vi "Grid ChangeValue.vi"(8 "error in (no error)":errorcluster caption="エラー入力（エラーなし）", 9 "OldVal":string[][](array[string]), 10 "NewVal":string[][](array[string]), 11 "出力クラスタ":T2) -> (0 "error out":errorcluster caption="エラー出力", 2 "編集位置":T1, 3 "変化位置配列":T1[](array[typedef]))   [LabVIEW 2014]
uses:
  <vilib>/Utility/miscctls.llb/LVRowAndColumnTypeDef.ctl
  Grid Parameter.ctl
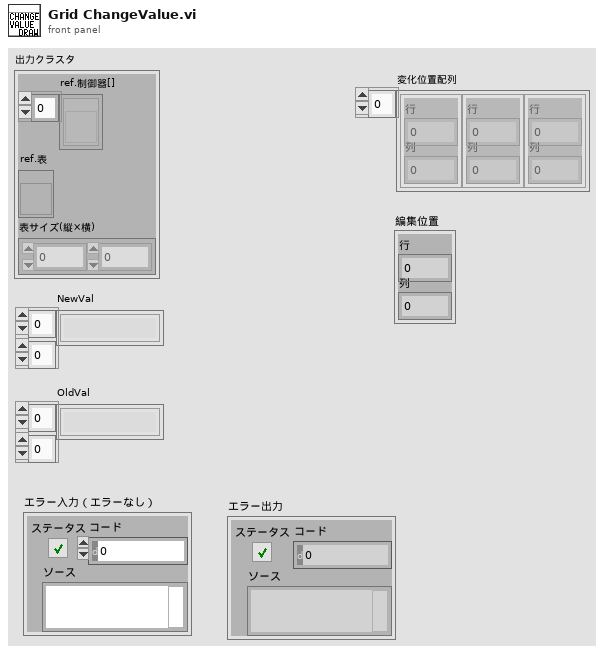
[diagram p1: front panel]
types:
  T1 = typedef "LVRowAndColumnTypeDef.ctl" = cluster{"Row":i32, "Column":i32}
  T2 = typedef "Grid Parameter.ctl" = cluster{"ref.制御器[]":refnum<vi>[], "ref.表":refnum<vi>, "表サイズ(縦×横)":i32[]}
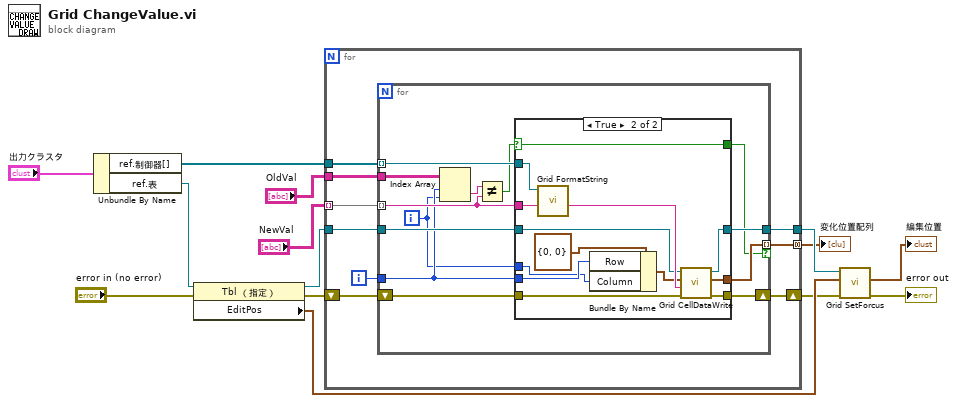
[diagram p0: block diagram]
diagram:
  n1 = Unbundle By Name("出力クラスタ") -> ("ref.制御器[]"=w2:refnum<vi>[], "ref.表"=w14:refnum<vi>)
  n2 = property class="Tbl （指定）"(reference=w14, error in="error in (no error)") -> (reference out=w10:refnum<vi>, error out=w1:errorcluster, "EditPos"=w12:T1)
  n3 = for {
    tunnel: "OldVal" -> [w23]
    tunnel: "NewVal" -> [w22] mode=indexing
    tunnel: w10 -> [w20]
    tunnel: [w19] -> w11
    shift-right: [w17] -> w6
    shift-left: w1 -> [w18]
    tunnel: [w16] -> w4 mode=concatenating
    tunnel: w2 -> [w15]
    i -> [w21]
    n4 = for {
      tunnel: w23 -> [w31]
      tunnel: w22 -> [w35] mode=indexing
      tunnel: w21 -> [w30]
      tunnel: w15 -> [w36] mode=indexing
      tunnel: w20 -> [w33]
      tunnel: [w32] -> w19
      shift-right: [w26] -> w17
      shift-left: w18 -> [w27]
      tunnel: [w25] -> w16 mode=indexing if=w24
      i -> [w29]
      n5 = Index Array(array=w31, index (row)=w30, index (col)=w29) -> (element=w28:string)
      n6 = Not Equal?(x=w28, y=w35) -> (x != y?=w34:bool)
      n7 = case shown="TRUE" w34 {
        selector: w34 -> [w37 w40]
        tunnel: w36 -> [_ w52]
        tunnel: w35 -> [_ w51]
        tunnel: w30 -> [_ w49]
        tunnel: w29 -> [_ w48]
        tunnel: w33 -> [w39 w45]
        tunnel: [w39 w44] -> w32
        tunnel: w27 -> [w38 w43]
        tunnel: [w38 w42] -> w26
        tunnel: [_ w41] -> w25
        tunnel: [w37 w40] -> w24
        frame False {
        }
        frame True {
          n8 = call "Grid FormatString.vi"("文字列"=w51, "Control入力"=w52) -> ("フォーマット後文字列"=w50:string)  [unwired: 9 in]
          n9 = Bundle By Name(cluster=T1 {"Row"=0, "Column"=0} ("EditPos"), "Row"=w49, "Column"=w48) -> (w46:T1)
          n10 = call "Grid CellDataWrite.vi"("error in (no error)"=w43, "RingText.Text"=w50, "EditPos"=w46, "Table入力"=w45) -> ("エラー出力"=w42:errorcluster, "EditPos(copy))"=w41:T1, "Table出力"=w44:refnum<vi>)  [unwired: 5 in]
        }
      }
    }
  }
  "変化位置配列" <- w4
  n11 = call "Grid SetForcus.vi"("エラー入力（エラーなし）"=w6, "EditPos入力"=w12, "Table入力"=w11) -> ("error out"=→"error out":errorcluster, "EditPos出力"=→"編集位置":T1)  [unwired: 6 in, 1 out]
